vi "Group Data Type.vi"(8 "error in (no error)":errorcluster, 11 "Group BOOL in":refnum<class "Group BOOL.lvclass">) -> (0 "error out":errorcluster, 2 "Group Data Type":T1, 3 "Group BOOL out":refnum<class "Group BOOL.lvclass">)   [LabVIEW 2020, in "Vecto.lvlib" / "Group BOOL.lvclass"]
uses:
  Group BOOL.lvclass
  Group BOOL.lvclass/Group BOOL.ctl
  Group Data Type.ctl
  VectoConfig/VectoConfig.lvlib
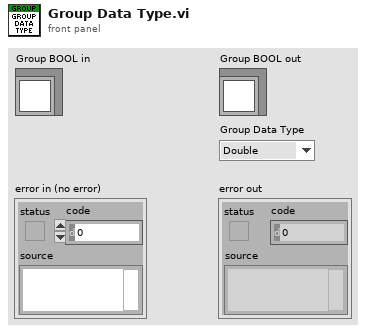
[diagram p1: front panel]
types:
  T1 = typedef "VectoConfig.lvlib/Group Data Type.ctl" = enum16{"Double", "String", "Bool"}
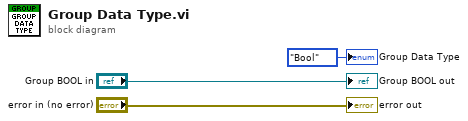
[diagram p0: block diagram]
diagram:
  "error out" <- "error in (no error)"
  "Group BOOL out" <- "Group BOOL in"
  "Group Data Type" <- Group_Data_Type."Bool" ("Group Data Type")
